vi "Psychrmoetric Chart by HR.vi"() -> (0 "Psych Chart by HR":dbl[][](array[numeric]))   [LabVIEW 2020]
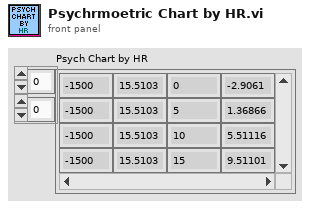
[diagram p1: front panel]
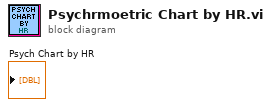
[diagram p0: block diagram]
diagram:
